vi "H5Lvisit.vi"(5 "Order":T1 items=["H5_ITER_UNKNOWN"=-1, "H5_ITER_INC"=0, "H5_ITER_DEC"=1], 6 "Callback VI Ref":refnum<vi>, 7 "Index Type":T2 items=["H5_INDEX_UNKNOWN"=-1, "H5_INDEX_NAME"=0, "H5_INDEX_CRT_ORDER"=1], 8 "error in (no error)":errorcluster, 10 "User data":variant, 11 "Location Ref":T3) -> (0 "error out":errorcluster, 2 "User data out":variant, 3 "Location Ref out":T3)   [LabVIEW 2017]
doc: "Recursively visits all links starting from a specified group."
uses:
  <vilib>/UPVI/lvhdf5/library.llb/HDF5 Ref.ctl
  <vilib>/UPVI/lvhdf5/library.llb/H5_index_t.ctl
  <vilib>/UPVI/lvhdf5/library.llb/H5_iter_order_t.ctl
panel:
  # "LVHDF5 Toolkit\nCopyright (c) 2005-2013 by Jason D. Sommerville\nCopyright (c) 2014-2015 by UPVI, LLC.\n\nThis use and distribution of this file is governed by the terms found in \nLICENSE.txt distributed with this toolkit and installed at\n <user.lib>\\_lvhdf5\\LICENSE.txt"
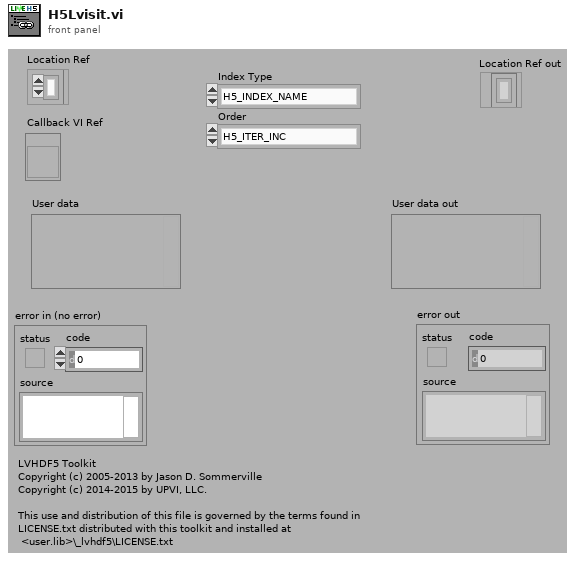
[diagram p1: front panel]
types:
  T1 = typedef "H5_iter_order_t.ctl" = i32
  T2 = typedef "H5_index_t.ctl" = i32
  T3 = typedef "HDF5 Ref.ctl" = refnum<k1>
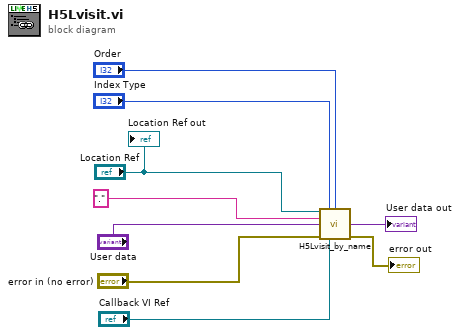
[diagram p0: block diagram]
diagram:
  n1 = call <vilib>:"H5Lvisit_by_name.vi"("Location Ref"="Location Ref", "Index Type"="Index Type", "Order"="Order", "Name"="." ("grp_name"), "User data"="User data", "error in (no error)"="error in (no error)", "Callback VI Ref"="Callback VI Ref") -> ("User data out"=→"User data out":variant, "error out"=→"error out":errorcluster)  [unwired: 6 in, 1 out]
  "Location Ref out" <- "Location Ref"
